vi "Test Noise Simulator.vi"() -> ()   [LabVIEW 2019, in "Instrument.Lockin.lvlib" / "Instrument.DAQ.lvclass"]
uses:
  Instrument.DAQ.lvclass
  DAQmx/DAQmx.lvclass
  Typedefs/DeviceInfo--Cluster.ctl
  Typedefs/DAQ.Sampling.Sampling--Cluster.ctl
  Typedefs/Simulation Mode--enum.ctl
  <vilib>/measure/NI_MABase.lvlib
  C:/Program Files/National Instruments/LabVIEW 2019/vi.lib/JKI/JKI SMO/SMO/SMO.lvclass
panel:
  out "Numeric":i32
  out "Noisy Signal Graph":waveform(dbl)[](graph)
  in  "stop":bool
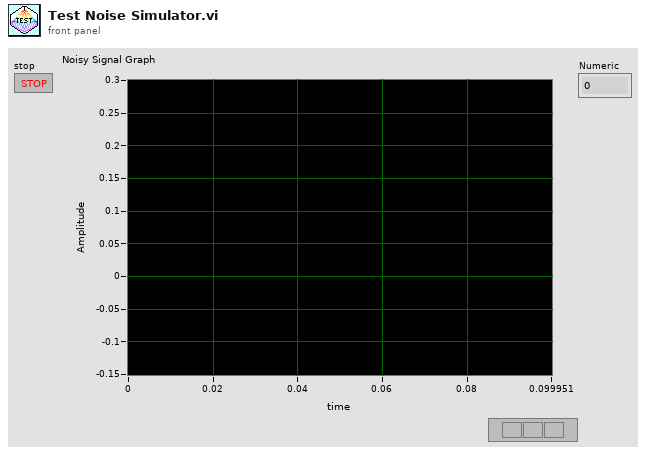
[diagram p1: front panel]
types:
  T1 = typedef "Instrument.Lockin.lvlib/Instrument.DAQ.lvclass/Simulation Mode--enum.ctl" = enum16{"AI = HW simulated", "AI = noise*AO", "AI = waveguide"}
  T2 = typedef "Instrument.Lockin.lvlib/Instrument.DAQ.lvclass/DAQ.Sampling.Sampling--Cluster.ctl" = cluster{"Fs":dbl, "#s":i32}
  T3 = typedef "Instrument.Lockin.lvlib/Instrument.DAQ.lvclass/DeviceInfo--Cluster.ctl" = cluster{"DeviceName":string, "DevIsSimulated":bool, "DeviceSerialNumber":string, "ProductType":string, "ProductCategory":i32, "ProductNumber":u32, "ChassisNumber":u32, "SlotNumber":u32, "ChassisName":string, "ChassisSerialNumber":string, "DevTemp":dbl, "SelfCal.LastDate/Time":string, "SelfCal.LastTemp":dbl, "calibration due?":bool}
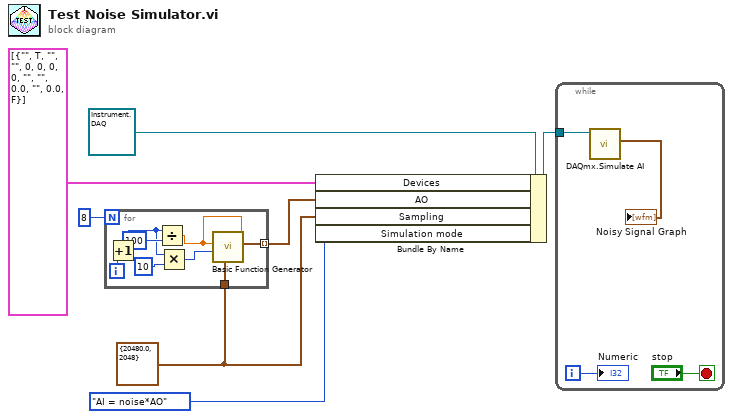
[diagram p0: block diagram]
diagram:
  w3 = T2 {"Fs"=20480.0, "#s"=2048} ("Configuration.DAQ.Sampling.Sampling")
  n1 = for {
    N: 8 -> [_]
    tunnel: w3 -> [w15]
    tunnel: [w14] -> w2 mode=indexing
    i -> [w13]
    n2 = Increment(x=w13) -> (x+1=w9:i32)
    n3 = Divide(x=w9, y=100) -> (x/y=w8:dbl)
    n4 = Multiply(x=w9, y=10) -> (x*y=w11:i32)
    n5 = call <vilib>:"Basic Function Generator.vi"("offset"=w8, "sampling info"=w15, "phase"=w11, "amplitude"=w8) -> ("signal out"=w14:waveform(dbl))  [unwired: 5 in, 2 out]
  }
  n6 = Bundle By Name(cluster=refnum<class "Instrument.DAQ.lvclass"> refnum ("Instrument.Lockin.lvlib:Instrument.DAQ.lvclass"), "Devices"=T3[] [{"DeviceName"="", "DevIsSimulated"=TRUE, "DeviceSerialNumber"="", "ProductType"="", "ProductCategory"=0, "ProductNumber"=0, "ChassisNumber"=0, "SlotNumber"=0, "ChassisName"="", "ChassisSerialNumber"="", "DevTemp"=0.0, "SelfCal.LastDate/Time"="", "SelfCal.LastTemp"=0.0, "calibration due?"=FALSE}] ("Configuration.DAQ.Devices"), "AO"=w2, "Sampling"=w3, "Simulation mode"=Simulation_Mode--enum."AI = noise*AO" ("Configuration.DAQ.Simulation mode")) -> (w6:refnum<class "Instrument.DAQ.lvclass">)
  n7 = while {
    tunnel: w6 -> [w19]
    i -> [w16]
    stop <- "stop" stop-if-true
    n8 = call "DAQmx.Simulate AI.vi"("DAQmx in"=w19) -> ("Noisy Signal Graph"=→"Noisy Signal Graph":waveform(dbl)[])  [unwired: 7 in, 3 out]
    "Numeric" <- w16
  }
